vi "Send Command.vi"(8 "error in (no error)":errorcluster, 10 "Command":string, 11 "VISA resource name":refnum<visa-resource-name>) -> (0 "error out":errorcluster, 2 "Read Value":string, 3 "VISA resource name out":refnum<visa-resource-name>)   [LabVIEW 2025, in "Interface Functions.lvlib"]
uses:
  Interface Functions.lvlib
  <vilib>/Utility/error.llb/Trim Whitespace One-Sided.vi
  <vilib>/Instr/_visa.llb/VISA Configure Serial Port (Instr).vi
  <vilib>/regexp/Match Regular Expression.xnode
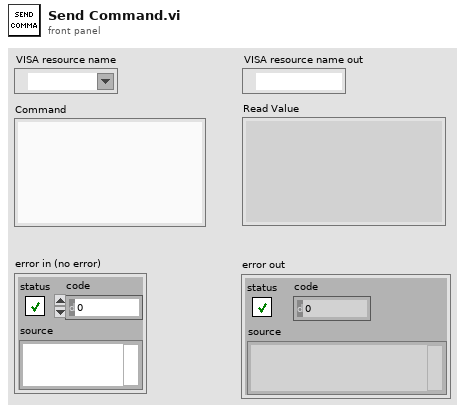
[diagram p1: front panel]
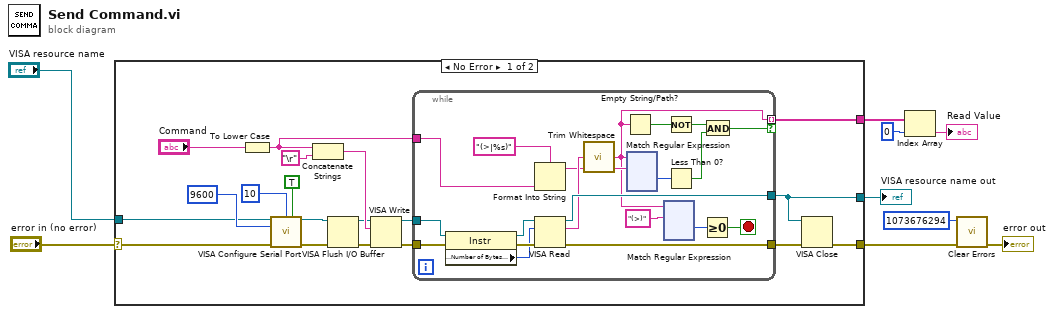
[diagram p0: block diagram]
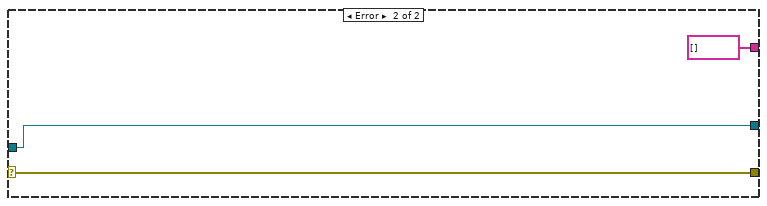
[diagram p2: hidden frame]
diagram:
  n1 = case shown="No Error" "error in (no error)" {
    selector: "error in (no error)" -> [w12 w285]
    tunnel: [w27 w285] -> w2
    tunnel: [w19 string[] []] -> w8
    tunnel: "VISA resource name" -> [w13 w283]
    tunnel: [w10 w283] -> w4
    frame No Error {
      n2 = To Lower Case(string="Command") -> (all lower case string=w14:string)
      n3 = call-poly "VISA Configure Serial Port"("VISA resource name"=w13, "termination char\n(0xA = '\\n' = LF)"=u8 10 ("termination char\n(0xA = '\\n' = LF)"), "Enable Termination\nChar (T)"=TRUE ("Enable Termination\nChar (T)"), "baud rate (9600)"=u32 9600, "error in (no error)"=w12) -> ("VISA resource name out"=w17:refnum<visa-resource-name>, "error out"=w18:errorcluster)  [unwired: 9 in]
      n4 = Concatenate Strings(w14, "\r") -> (w23:string)
      n5 = VISA Flush I/O Buffer(VISA resource name=w17, error in (no error)=w18) -> (VISA resource name out=w15:refnum<visa-resource-name>, error out=w16:errorcluster)  [unwired: 1 in]
      n6 = VISA Write(VISA resource name=w15, write buffer=w23, error in (no error)=w16) -> (VISA resource name out=w21:refnum<visa-resource-name>, error out=w20:errorcluster)  [unwired: 1 out]
      n7 = while {
        tunnel: w20 -> [w42]
        tunnel: [w44] -> w25
        tunnel: w21 -> [w43]
        tunnel: [w45] -> w10
        tunnel: [w33] -> w19 mode=indexing if=w29
        tunnel: w14 -> [w35]
        stop <- w39 stop-if-true
        n8 = property class="Instr"(reference=w43, error in=w42) -> (reference out=w46:refnum<visa-resource-name>, error out=w48:errorcluster, "Serial Settings:Number of Bytes at Serial Port"=w47:u32)
        n9 = Format Into String(format string="(>|%s)" ("regular expression"), w35) -> (resulting string=w34:string)  [unwired: 2 in, 1 out]
        n10 = VISA Read(VISA resource name=w46, byte count=w47, error in (no error)=w48) -> (VISA resource name out=w45:refnum<visa-resource-name>, read buffer=w41:string, error out=w44:errorcluster)  [unwired: 1 out]
        n11 = call <vilib>:"Trim Whitespace.vi"("string"=w41) -> ("trimmed string"=w33:string)  [unwired: 1 in]
        n12 = Empty String/Path?(string/path=w33) -> (empty?=w37:bool)
        n13 = xnode "Match Regular Expression"("input string"=w33, "regular expression"=w34) -> ("offset past match"=w31:i32)  [unwired: 4 in, 4 out]
        n14 = xnode "Match Regular Expression"("input string"=w33, "regular expression"="(>)") -> ("offset past match"=w40:i32)  [unwired: 4 in, 4 out]
        n15 = Not(x=w37) -> (.not. x?=w32:bool)
        n16 = Less Than 0?(x=w31) -> (x < 0?=w30:bool)
        n17 = Greater Or Equal To 0?(x=w40) -> (x >= 0?=w39:bool)
        n18 = And(x=w32, y=w30) -> (x .and. y?=w29:bool)
      }
      n19 = VISA Close(VISA resource name=w10, error in (no error)=w25) -> (error out=w27:errorcluster)
    }
    frame Error {
    }
  }
  "VISA resource name out" <- w4
  n20 = Index Array(array=w8, index=0) -> (element=→"Read Value":string)
  n21 = call <vilib>:"Clear Errors.vi"("error in (no error)"=w2, "specific error code to clear (0: all)"=1073676294) -> ("error out"=→"error out":errorcluster)  [unwired: 4 in, 1 out]
